vi "Example files directory.vi"(7 "File Type":enum16{"DXF", "GCODE"}(ring)) -> (3 "path":path)   [LabVIEW 2014]
doc: "Get the dir path of the example DXF and GCODE files."
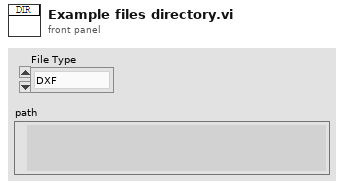
[diagram p1: front panel]
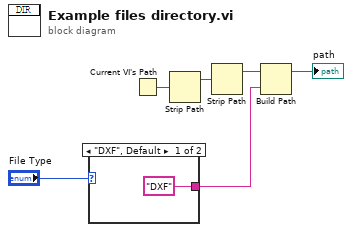
[diagram p0: block diagram]
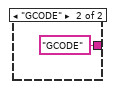
[diagram p2: hidden frame]
diagram:
  n1 = case shown="\"DXF\", Default" "File Type" {
    tunnel: ["DXF" "GCODE"] -> w1
    frame "DXF", Default {
    }
    frame "GCODE" {
    }
  }
  n2 = Current VI's Path() -> (path=w6:path)
  n3 = Strip Path(path=w6) -> (stripped path=w5:path)  [unwired: 1 out]
  n4 = Strip Path(path=w5) -> (stripped path=w4:path)  [unwired: 1 out]
  n5 = Build Path(base path=w4, name or relative path=w1) -> (appended path=→"path":path)
